vi "RecieveACmd.vi"(11 "Digit Signal":bool) -> (0 "Error?":bool, 1 "Finished?":bool, 3 "Cmd":u8[](array[numeric]))   [LabVIEW 2013]
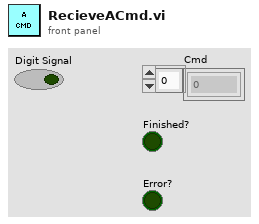
[diagram p1: front panel]
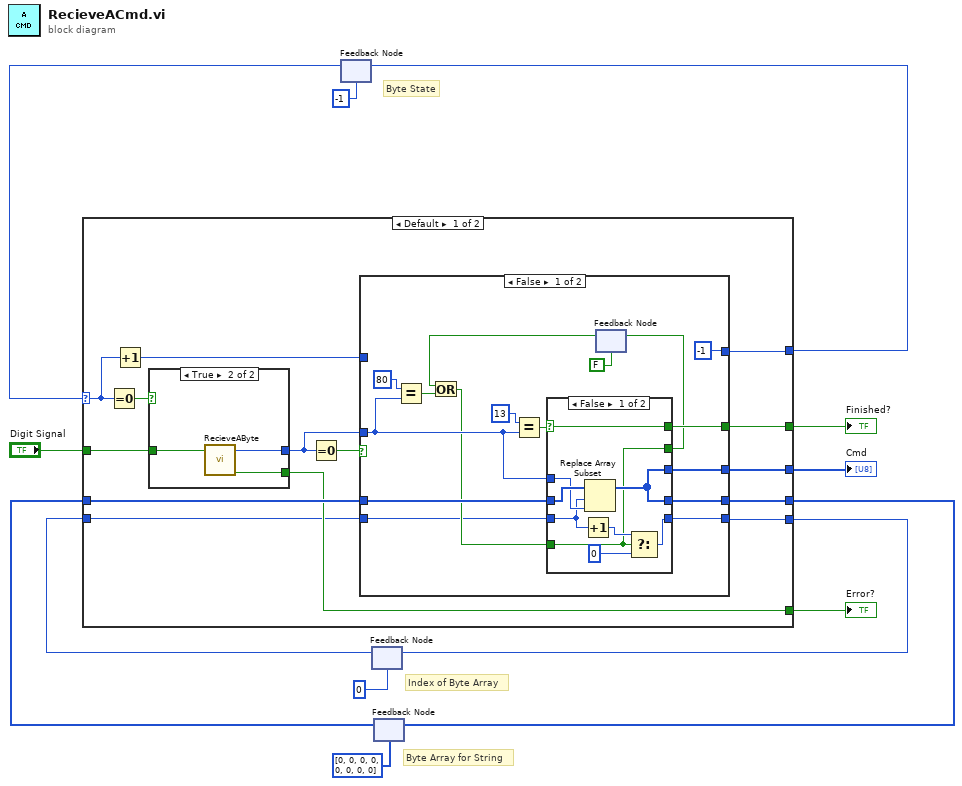
[diagram p0: block diagram]
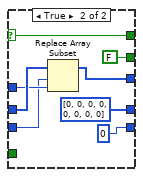
[diagram p2: hidden frame]
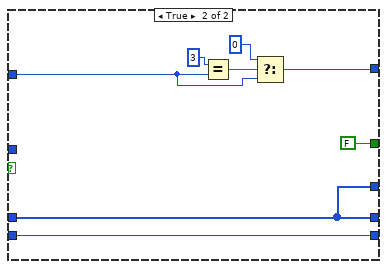
[diagram p3: hidden frame]
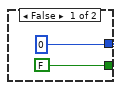
[diagram p4: hidden frame]
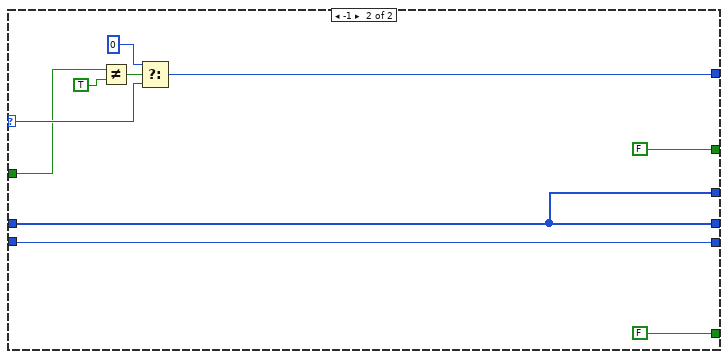
[diagram p5: hidden frame]
diagram:
  # "Byte Array for String"
  # "Index of Byte Array"
  # "Byte State"
  n1 = feedback #1(i8 -1) -> (w11:i32)
  n2 = feedback #2(u8 0) -> (w2:u8)
  n3 = feedback #3(u8[] [0, 0, 0, 0, 0, 0, 0, 0]) -> (w9:u8[])
  n4 = case shown="Default" w11 {
    selector: w11 -> [w14 w79]
    tunnel: "Digit Signal" -> [w27 w78]
    tunnel: [w25 w80] -> w10
    tunnel: w9 -> [w24 w76]
    tunnel: [w23 w76] -> w8
    tunnel: [w22 FALSE] -> w7
    tunnel: [w21 w76] -> w5
    tunnel: [w20 FALSE] -> w4
    tunnel: w2 -> [w17 w74]
    tunnel: [w16 w74] -> w1
    frame Default {
      n5 = Equal To 0?(x=w14) -> (x = 0?=w15:bool)
      n6 = Increment(x=w14) -> (x+1=w26:i32)
      n7 = case shown="True" w15 {
        tunnel: w27 -> [_ w73]
        tunnel: [u8 0 w71] -> w18
        tunnel: [FALSE w72] -> w20
        frame False {
        }
        frame True {
          n8 = call "RecieveAByte.vi"("Digit Signal"=w73) -> ("Error?"=w72:bool, "Char"=w71:u8)  [unwired: 9 in]
        }
      }
      n9 = Equal To 0?(x=w18) -> (x = 0?=w19:bool)
      n10 = case shown="False" w19 {
        tunnel: w26 -> [_ w61]
        tunnel: [-1 w64] -> w25
        tunnel: w18 -> [w34 _]
        tunnel: w24 -> [w42 w67]
        tunnel: [w39 w67] -> w23
        tunnel: [w41 FALSE] -> w22
        tunnel: [w40 w67] -> w21
        tunnel: w17 -> [w28 w66]
        tunnel: [w38 w66] -> w16
        frame False {
          n11 = Equal?(x=u8 80, y=w34) -> (x = y?=w32:bool)
          n12 = Equal?(x=u8 13, y=w34) -> (x = y?=w37:bool)
          n13 = feedback #4(FALSE) -> (w31:bool)
          n14 = Or(x=w31, y=w32) -> (x .or. y?=w29:bool)
          n15 = case shown="False" w37 {
            selector: w37 -> [w52 w60]
            tunnel: w42 -> [w51 w57]
            tunnel: w34 -> [w50 w55]
            tunnel: [w52 w60] -> w41
            tunnel: [w49 w56] -> w40
            tunnel: [w49 u8[] [0, 0, 0, 0, 0, 0, 0, 0]] -> w39
            tunnel: [w46 u8 0] -> w38
            tunnel: [w45 FALSE] -> w30
            tunnel: w29 -> [w45 _]
            tunnel: w28 -> [w44 w53]
            frame False {
              n16 = Increment(x=w44) -> (x+1=w48:u8)
              n17 = Replace Array Subset(array=w51, new element=w50, index=w44) -> (w49:u8[])
              n18 = Select(t=w48, s=w45, f=u8 0) -> (s? t:f=w46:u8)
            }
            frame True {
              n19 = Replace Array Subset(array=w57, new element=w55, index=w53) -> (w56:u8[])
            }
          }
          n20 = feedback-in #4(w30) -> ()
        }
        frame True {
          n21 = Equal?(x=i8 3, y=w61) -> (x = y?=w65:bool)
          n22 = Select(t=i8 0, s=w65, f=w61) -> (s? t:f=w64:i32)
        }
      }
    }
    frame -1 {
      n23 = Not Equal?(x=w78, y=TRUE) -> (x != y?=w82:bool)
      n24 = Select(t=i8 0, s=w82, f=w79) -> (s? t:f=w80:i32)
    }
  }
  "Finished?" <- w7
  "Cmd" <- w5
  "Error?" <- w4
  n25 = feedback-in #1(w10) -> ()
  n26 = feedback-in #2(w1) -> ()
  n27 = feedback-in #3(w8) -> ()
